vi "Set UUT Test Result.vi"(0 "reference in":refnum<class "UUT.lvclass">, 1 "Push Values (lb)":dbl[](array[numeric]), 2 "Push Average (lb)":dbl, 3 "Push Std Dev (lb)":dbl, 4 "Pull Values (lb)":dbl[](array[numeric]), 5 "Pull Average (lb)":dbl, 6 "Pull Std Dev (lb)":dbl, 7 "error in (no error)":errorcluster) -> (20 "reference out":refnum<class "UUT.lvclass">, 27 "error out":errorcluster)   [LabVIEW 2017, in "UUT.lvclass"]
uses:
  UUT.lvclass
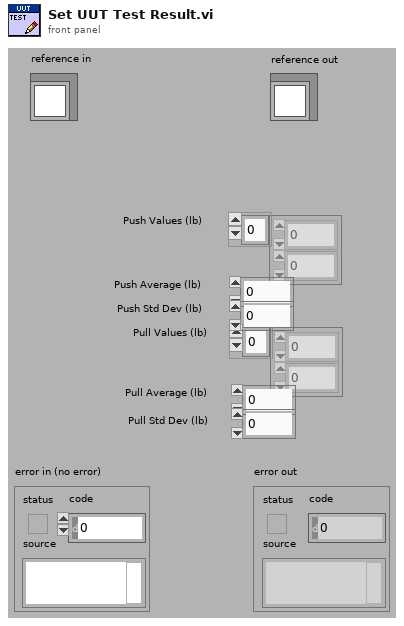
[diagram p1: front panel]
types:
  T1 = typedef "UUT.lvclass/ObjectAttributes.ctl" = cluster{"UUT Info":cluster{"Part Number":string, "Lower Push Limit (lb)":dbl, "Upper Push Limit (lb)":dbl, "Lower Pull Limit (lb)":dbl, "Upper Pull Limit (lb)":dbl, "Push Position (mm)":dbl, "Pull Position (mm)":dbl}, "Test Results":cluster{"Test Time":timestamp, "Number of Trials":u32, "Push Values (lb)":dbl[], "Push Average (lb)":dbl, "Push Std Dev (lb)":dbl, "Push Passed":bool, "Pull Values (lb)":dbl[], "Pull Average (lb)":dbl, "Pull Std Dev (lb)":dbl, "Pull Passed":bool}}
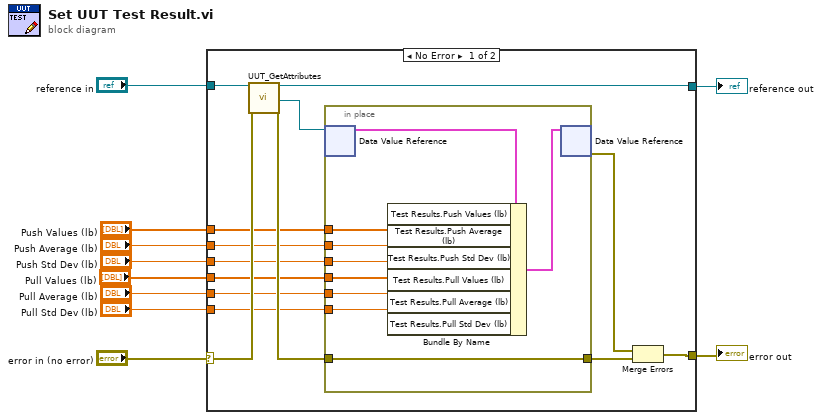
[diagram p0: block diagram]
diagram:
  n1 = case shown="No Error" "error in (no error)" {
    selector: "error in (no error)" -> [w23 w35]
    tunnel: [w20 w35] -> w9
    tunnel: [w21 w34] -> w7
    tunnel: "reference in" -> [w24 w34]
    tunnel: "Pull Std Dev (lb)" -> [w16 _]
    tunnel: "Pull Average (lb)" -> [w15 _]
    tunnel: "Pull Values (lb)" -> [w14 _]
    tunnel: "Push Std Dev (lb)" -> [w13 _]
    tunnel: "Push Average (lb)" -> [w12 _]
    tunnel: "Push Values (lb)" -> [w11 _]
    frame No Error {
      n2 = call "UUT_GetAttributes.vi"("reference in"=w24, "error in (no error)"=w23) -> ("reference out"=w21:refnum<class "UUT.lvclass">, "DataRef"=w19:refnum<data-value>, "error out"=w18:errorcluster)  [unwired: 14 in, 1 out]
      n3 = in-place {
        in-place-border: w18 -> [w33]
        in-place-border: [w33] -> w17
        in-place-border: w16 -> [w25]
        in-place-border: w15 -> [w26]
        in-place-border: w14 -> [w27]
        in-place-border: w13 -> [w28]
        in-place-border: w12 -> [w29]
        in-place-border: w11 -> [w30]
        n4 = in-place-dvr #1(w19) -> (w32:T1)  [unwired: 1 out]
        n5 = Bundle By Name(cluster=w32, "Test Results.Push Values (lb)"=w30, "Test Results.Push Average (lb)"=w29, "Test Results.Push Std Dev (lb)"=w28, "Test Results.Pull Values (lb)"=w27, "Test Results.Pull Average (lb)"=w26, "Test Results.Pull Std Dev (lb)"=w25) -> (w31:T1)
        n6 = in-place-dvr #1(w31) -> (w22:errorcluster)  [unwired: 1 out]
      }
      n7 = Merge Errors(w22, w17) -> (w20:errorcluster)
    }
    frame Error {
    }
  }
  "error out" <- w9
  "reference out" <- w7
